vi "Add Target_Add Target.vi"(8 "error in (no error)":errorcluster, 10 "Settings":T1={"Name"="", "Target Type"="", "IPAddress"="localhost", "PrimaryControlLoopProcessor"=-2, "DataProcessingLoopProcessor"=-2, "DataProcessingLoopDecimation"=1, "DAQDigitalLinesDecimation"=1, "MaximumStreamedChannels"=512, "ExecutionMode"=0, "FilterDAQErrors"=FALSE, "FilterWatchdogErrors"=FALSE, "FPGAScanInterfaceMode"=0, "TargetRate"=0.0} {"FPGAScanInterfaceMode" items=["Use Current", "FPGA Mode", "Scan Mode"]; "ExecutionMode" items=["Parallel", "LowLatency"]}, 11 "Targets Ref":refnum<k24>) -> (0 "error out":errorcluster, 2 "Target Reference":refnum<k24>)   [LabVIEW 2019, in "Simple SysDef API.lvlib"]
uses:
  <userlib>/SimpleSysDef/Simple SysDef API.lvlib
  <userlib>/SimpleSysDef/_SubVIs/Add Target_Settings.ctl
  <userlib>/SimpleSysDef/_SubVIs/Add Target_Types.ctl
  NationalInstruments.VeriStand.SystemDefinitionAPI
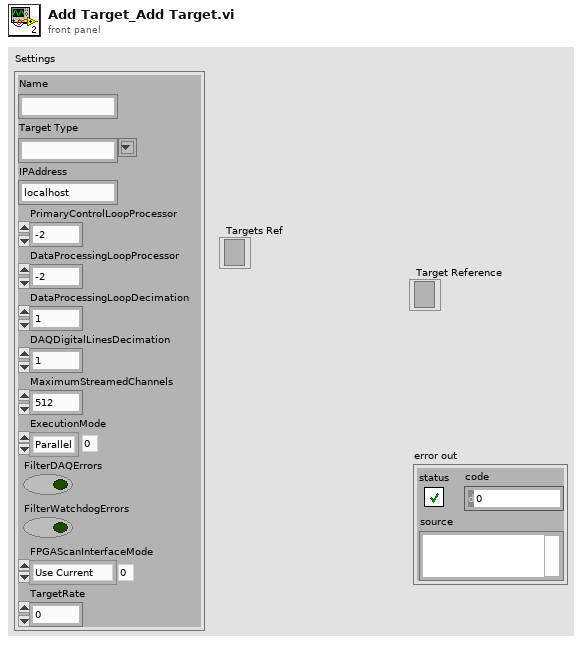
[diagram p1: front panel]
types:
  T1 = typedef "Simple SysDef API.lvlib/Add Target_Settings.ctl" = cluster{"Name":string, "Target Type":T2, "IPAddress":string, "PrimaryControlLoopProcessor":i32, "DataProcessingLoopProcessor":i32, "DataProcessingLoopDecimation":i32, "DAQDigitalLinesDecimation":u32, "MaximumStreamedChannels":i32, "ExecutionMode":i32, "FilterDAQErrors":bool, "FilterWatchdogErrors":bool, "FPGAScanInterfaceMode":u16, "TargetRate":dbl}
  T2 = typedef "Simple SysDef API.lvlib/Add Target_Types.ctl" = string
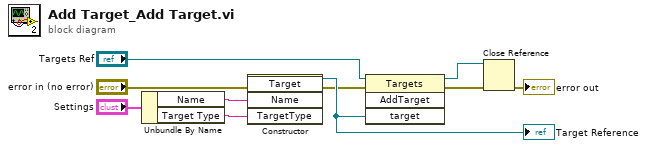
[diagram p0: block diagram]
diagram:
  n1 = Unbundle By Name("Settings") -> ("Name"=w8:string, "Target Type"=w7:T2)
  n2 = constructor class="Target"(error in="error in (no error)", "Name"=w8, "TargetType"=w7) -> (reference out=w5:refnum<k24>, error out=w4:errorcluster)  [unwired: 2 in, 3 out]
  "Target Reference" <- w5
  n3 = invoke class="Targets" method="AddTarget"(reference="Targets Ref", error in=w4, "target"=w5) -> (reference out=w1:refnum<k24>, error out=w3:errorcluster)  [unwired: 1 in, 2 out]
  n4 = Close Reference(reference=w1, error in (no error)=w3) -> (error out=→"error out":errorcluster)
